vi "Read XML Parameters File_Parse Read Data.vi"(6 "Close Ref?":bool=TRUE, 8 "error in (no error)":errorcluster, 11 ".NET Refnum in":refnum<k24>) -> (0 "error out":errorcluster, 2 ".NET Refnum out":refnum<k24>, 3 "Channels":T1[](array[typedef]))   [LabVIEW 2019]
uses:
  XML_Channel.ctl
  XML_Label.ctl
  XML_Parameter.ctl
  C:/Users/Localization Tester/Desktop/GIT/Ballard-Arinc-429-Custom-Device/Source/System Explorer/SubVIs/Parse Parameters File/Parameters_Arinc429_XML_Tools.dll
  Parameters_Arinc429_XML_Tools.dll
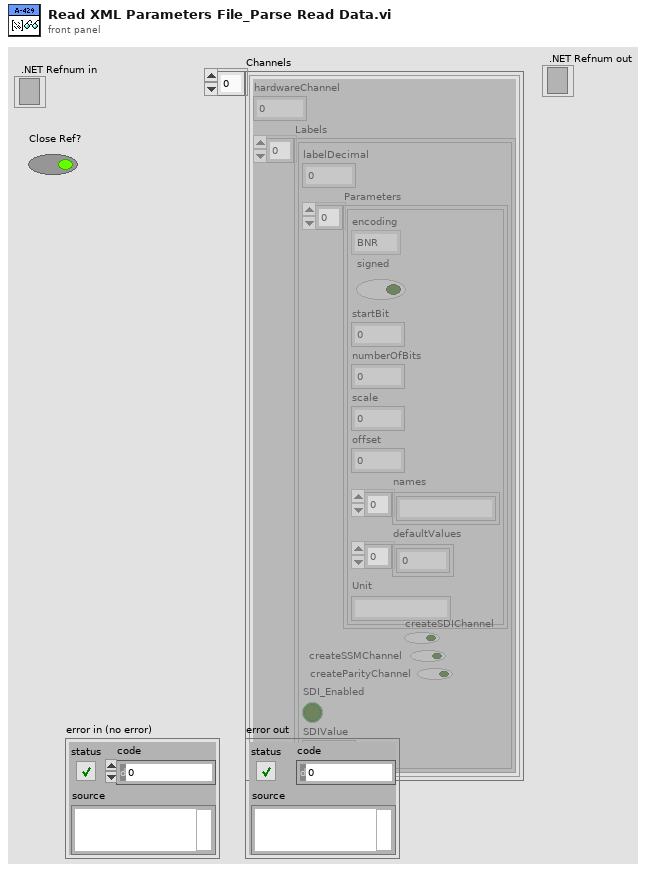
[diagram p1: front panel]
types:
  T1 = typedef "XML_Channel.ctl" = cluster{"hardwareChannel":i32, "Labels":T2[]}
  T2 = typedef "XML_Label.ctl" = cluster{"labelDecimal":i32, "Parameters":T3[], "createSDIChannel":bool, "createSSMChannel":bool, "createParityChannel":bool, "SDI_Enabled":bool, "SDIValue":u8}
  T3 = typedef "XML_Parameter.ctl" = cluster{"encoding":enum16{"BNR", "BCD", "Discrete"}, "signed":bool, "startBit":i32, "numberOfBits":i32, "scale":dbl, "offset":dbl, "names":string[], "defaultValues":dbl[], "Unit":string}
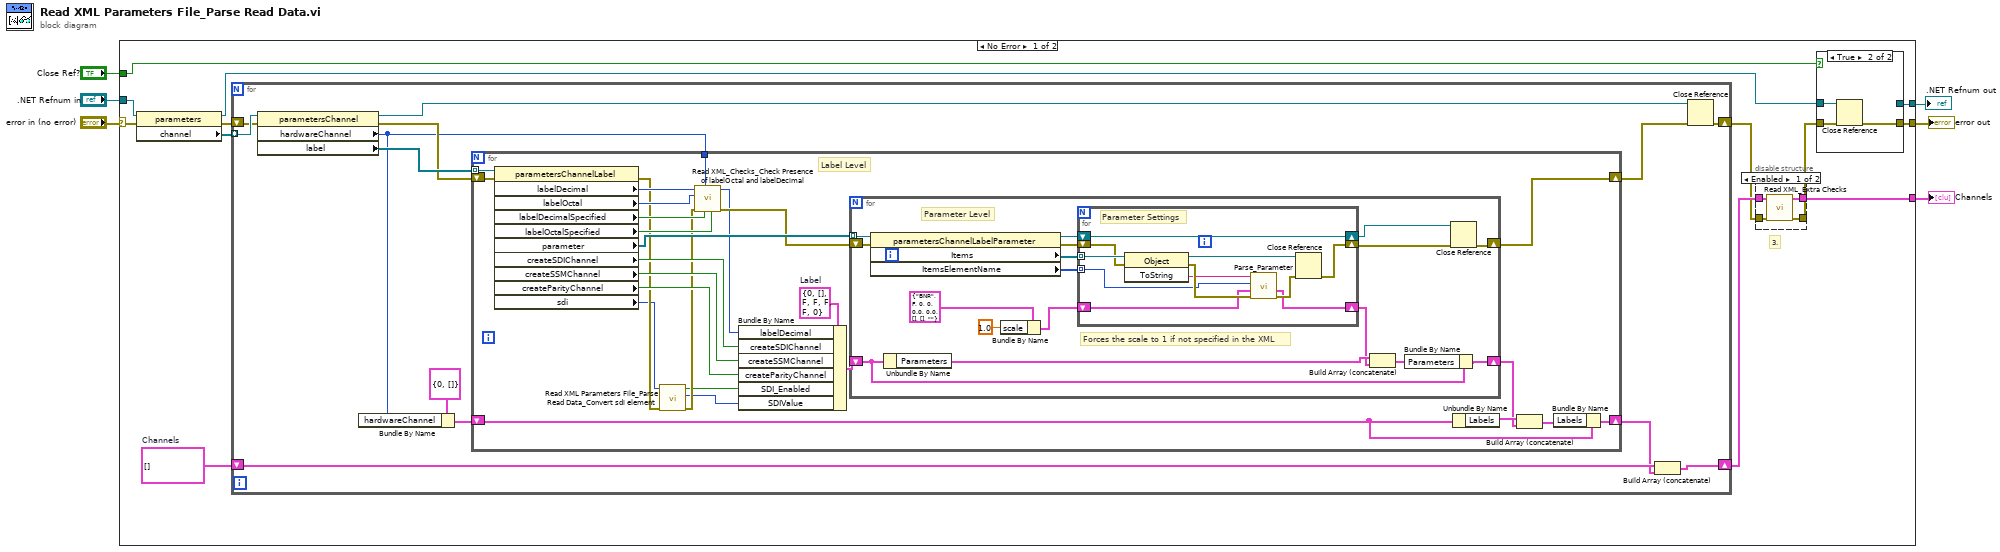
[diagram p0: block diagram]
diagram:
  n1 = case shown="No Error" "error in (no error)" {
    selector: "error in (no error)" -> [w9 w98]
    tunnel: [w17 _] -> w6
    tunnel: ".NET Refnum in" -> [w11 _]
    tunnel: [w10 w98] -> w4
    tunnel: "Close Ref?" -> [w8 _]
    tunnel: [w7 _] -> w1
    frame No Error {
      w18 = T1[] []  # Channels
      # "3."
      n2 = property class="parameters"(reference=w11, error in=w9) -> (reference out=w13:refnum<k24>, error out=w14:errorcluster, "channel"=w12:refnum<k24>[])
      n3 = for {
        tunnel: w12 -> [w43] mode=indexing
        shift-right: [w40] -> w15
        shift-left: w14 -> [w42]
        shift-right: [w33] -> w19
        shift-left: w18 -> [w34]
        n4 = property class="parametersChannel"(reference=w43, error in=w42) -> (reference out=w41:refnum<k24>, error out=w38:errorcluster, "hardwareChannel"=w31:i32, "label"=w39:refnum<k24>[])
        n5 = Bundle By Name(cluster=T1 {"hardwareChannel"=0, "Labels"=[]} ("Channel"), "hardwareChannel"=w31) -> (w35:T1)
        n6 = for {
          tunnel: w39 -> [w69] mode=indexing
          shift-right: [w66] -> w37
          shift-left: w38 -> [w68]
          shift-right: [w59] -> w32
          shift-left: w35 -> [w61]
          tunnel: w31 -> [w49]
          w65 = T2 {"labelDecimal"=0, "Parameters"=[], "createSDIChannel"=FALSE, "createSSMChannel"=FALSE, "createParityChannel"=FALSE, "SDI_Enabled"=FALSE, "SDIValue"=0}  # Label
          # "Label Level"
          n7 = property class="parametersChannelLabel"(reference=w69, error in=w68) -> (error out=w48:errorcluster, "labelDecimal"=w53:i32, "labelOctal"=w52:i32, "labelDecimalSpecified"=w51:bool, "labelOctalSpecified"=w50:bool, "parameter"=w67:refnum<k24>[], "createSDIChannel"=w58:bool, "createSSMChannel"=w57:bool, "createParityChannel"=w56:bool, "sdi"=w46:i32)  [unwired: 1 out]
          n8 = call "Read XML Parameters File_Parse Read Data_Convert sdi element.vi"("error in (no error)"=w48, "sdi"=w46) -> ("error out"=w47:errorcluster, "SDIValue"=w44:u8, "SDI_Enabled"=w45:bool)  [unwired: 7 in]
          n9 = call "Read XML_Checks_Check Presence of labelOctal and labelDecimal.vi"("labelOctalSpecified"=w50, "labelDecimalSpecified"=w51, "hardwareChannel"=w49, "error in (no error)"=w47, "labelOctal"=w52, "labelDecimal"=w53) -> ("error out"=w55:errorcluster, "labelDecimal"=w54:i32)  [unwired: 4 in]
          n10 = Bundle By Name(cluster=w65, "labelDecimal"=w54, "createSDIChannel"=w58, "createSSMChannel"=w57, "createParityChannel"=w56, "SDI_Enabled"=w45, "SDIValue"=w44) -> (w64:T2)
          n11 = for {
            tunnel: w67 -> [w85] mode=indexing
            shift-right: [w80] -> w66
            shift-left: w55 -> [w86]
            shift-right: [w76] -> w62
            shift-left: w64 -> [w77]
            # "Forces the scale to 1 if not specified in the XML"
            # "Parameter Level"
            n12 = property class="parametersChannelLabelParameter"(reference=w85, error in=w86) -> (reference out=w84:refnum<k24>, error out=w83:errorcluster, "Items"=w79:refnum<k24>[], "ItemsElementName"=w78:i32[])
            n13 = Unbundle By Name(w77) -> ("Parameters"=w75:T3[])
            n14 = Bundle By Name(cluster=T3 {"encoding"=enum."BNR", "signed"=FALSE, "startBit"=0, "numberOfBits"=0, "scale"=0.0, "offset"=0.0, "names"=[], "defaultValues"=[], "Unit"=""} ("Parameter"), "scale"=1.0) -> (w71:T3)
            n15 = for {
              shift-right: [w96] -> w82
              shift-left: w83 -> [w94]
              shift-right: [w97] -> w81
              shift-left: w84 -> [w97]
              tunnel: w79 -> [w95] mode=indexing
              tunnel: w78 -> [w87] mode=indexing
              shift-right: [w88] -> w73
              shift-left: w71 -> [w89]
              # "Parameter Settings"
              n16 = invoke class="Object" method="ToString"(reference=w95, error in=w94) -> (reference out=w93:refnum<k24>, error out=w92:errorcluster, "ToString"=w90:string)  [unwired: 1 in]
              n17 = call "Parse_Parameter.vi"("error in (no error)"=w92, "Parameter In"=w89, "ItemName"=w87, "Value (String)"=w90) -> ("error out"=w91:errorcluster, "Parameter Out"=w88:T3)  [unwired: 6 in]
              n18 = Close Reference(reference=w93, error in (no error)=w91) -> (error out=w96:errorcluster)
            }
            n19 = Build Array (concatenate)(w75, w73) -> (w74:T3[])
            n20 = Bundle By Name(cluster=w77, "Parameters"=w74) -> (w76:T2)
            n21 = Close Reference(reference=w81, error in (no error)=w82) -> (error out=w80:errorcluster)
          }
          n22 = Unbundle By Name(w61) -> ("Labels"=w63:T2[])
          n23 = Build Array (concatenate)(w63, w62) -> (w60:T2[])
          n24 = Bundle By Name(cluster=w61, "Labels"=w60) -> (w59:T1)
        }
        n25 = Build Array (concatenate)(w34, w32) -> (w33:T1[])
        n26 = Close Reference(reference=w41, error in (no error)=w37) -> (error out=w40:errorcluster)
      }
      n27 = disable-structure shown="Enabled" {
        disable-tunnel: w15 -> [w28 w30]
        disable-tunnel: [w27 w30] -> w16
        disable-tunnel: [w26 w29] -> w17
        disable-tunnel: w19 -> [w25 w29]
        frame Enabled {
          n28 = call "Read XML_Extra Checks.vi"("error in (no error)"=w28, "Channels In"=w25) -> ("error out"=w27:errorcluster, "Channels Out"=w26:T1[])  [unwired: 8 in]
        }
        frame Disabled {
        }
      }
      n29 = case shown="True" w8 {
        tunnel: w16 -> [w21 w24]
        tunnel: w13 -> [w20 w23]
        tunnel: [w21 w22] -> w10
        tunnel: [w20 _] -> w7
        frame False {
        }
        frame True {
          n30 = Close Reference(reference=w23, error in (no error)=w24) -> (error out=w22:errorcluster)
        }
      }
    }
    frame Error {
    }
  }
  "Channels" <- w6
  "error out" <- w4
  ".NET Refnum out" <- w1
